vi "Paths.vi"() -> (3 "Paths":T1)   [LabVIEW 2020, in "Summer of LabVIEW.lvlib" / "SOL-Server.lvclass"]
uses:
  SOL-Server.lvclass
  Paths.ctl
  SOL-Server.lvclass/SOL-Server.ctl
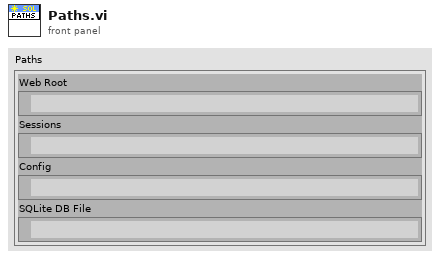
[diagram p1: front panel]
types:
  T1 = typedef "Summer of LabVIEW.lvlib/SOL-Server.lvclass/Paths.ctl" = cluster{"Web Root":path, "Sessions":path, "Config":path, "SQLite DB File":path}
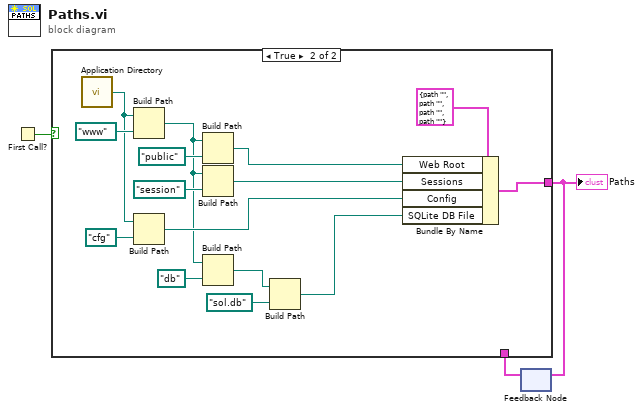
[diagram p0: block diagram]
diagram:
  n1 = First Call?() -> (First Call?: T/F=w1:bool)
  n2 = feedback #1() -> (w2:T1)  [unwired: 1 in]
  n3 = case shown="True" w1 {
    tunnel: [w4 w11] -> w3
    tunnel: w2 -> [w4 _]
    frame False {
    }
    frame True {
      n4 = call <vilib>:"Application Directory.vi"() -> ("Application Directory"=w5:path)
      n5 = Build Path(base path=w5, name or relative path=path "www") -> (appended path=w6:path)
      n6 = Build Path(base path=w5, name or relative path=path "cfg") -> (appended path=w12:path)
      n7 = Build Path(base path=w6, name or relative path=path "public") -> (appended path=w13:path)
      n8 = Build Path(base path=w6, name or relative path=path "session") -> (appended path=w14:path)
      n9 = Build Path(base path=w6, name or relative path=path "db") -> (appended path=w8:path)
      n10 = Build Path(base path=w8, name or relative path=path "sol.db") -> (appended path=w7:path)
      n11 = Bundle By Name(cluster=T1 {"Web Root"=path "", "Sessions"=path "", "Config"=path "", "SQLite DB File"=path ""} ("Paths"), "Web Root"=w13, "Sessions"=w14, "Config"=w12, "SQLite DB File"=w7) -> (w11:T1)
    }
  }
  "Paths" <- w3
  n12 = feedback-in #1(w3) -> ()
